vi "Teleop.vi"(10 "Match Info":T1={"Autonomous Elapsed Seconds"=0.0, "TeleOp Elapsed Seconds"=0.0, "Disabled Elapsed Seconds"=0.0, "Visited Autonomous"=FALSE, "Visited TeleOp"=FALSE, "Visited Disabled"=FALSE, "Autonomous Settings"={"Autonomous Style"=enum."Independent", "VI Refnum"=refnum}}, 11 "Call Context":T2) -> ()   [LabVIEW 2014]
doc: "This VI is called for each TeleOp packet received from the DS where the robot is not disabled. It is often used to read from the joysticks and update I/O or to update setpoints for timed control loops. It should complete and return within 20 milliseconds or it may miss DS packets."
uses:
  <vilib>/Rock Robotics/WPI/DriverStation/WPI_DriverStationDerivedRobotMode.ctl
  <vilib>/Rock Robotics/WPI/DriverStation/WPI_DriverStationMatch Info.ctl
  <vilib>/Rock Robotics/WPI/Joystick/WPI_JoystickGetSetRefNum.vi
  Robot Global Data.vi
panel:
  out "Operator Buttons":bool[](array[boolean])
  out "Driver Axis":dbl[](array[numeric])
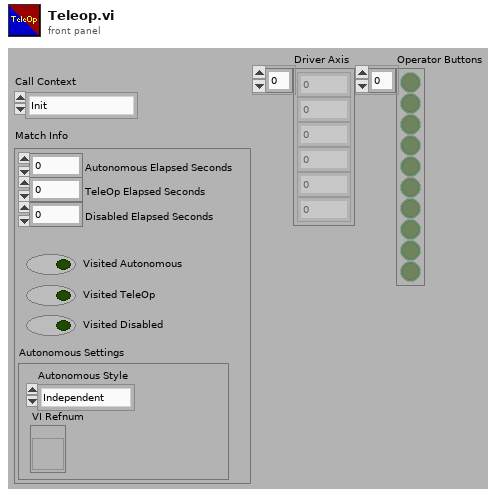
[diagram p1: front panel]
types:
  T1 = typedef "WPI_DriverStationMatch Info.ctl" = cluster{"Autonomous Elapsed Seconds":dbl, "TeleOp Elapsed Seconds":dbl, "Disabled Elapsed Seconds":dbl, "Visited Autonomous":bool, "Visited TeleOp":bool, "Visited Disabled":bool, "Autonomous Settings":cluster{"Autonomous Style":enum16{"Iterative", "Independent"}, "VI Refnum":refnum<vi>}}
  T2 = typedef "WPI_DriverStationDerivedRobotMode.ctl" = enum16{"Init", "Execute", "Stop"}
  T3 = typedef "WPI_JoystickDevRef.ctl" = cluster{"Device":T4}
  T4 = typedef "WPI_JoystickDeviceEnum.ctl" = enum16{"USB 0", "USB 1", "USB 2", "USB 3", "USB 4", "USB 5"}
  T5 = cluster{"String Potentiometer":dbl, "Setpoint":dbl, "Level":sgl}
  T6 = cluster{"Motor Speed":dbl, "Grabber":bool, "Brake":bool, "Trying To Brake":bool}
  T7 = cluster{"Lifter":bool, "Infeeds On":bool, "Descender":bool}
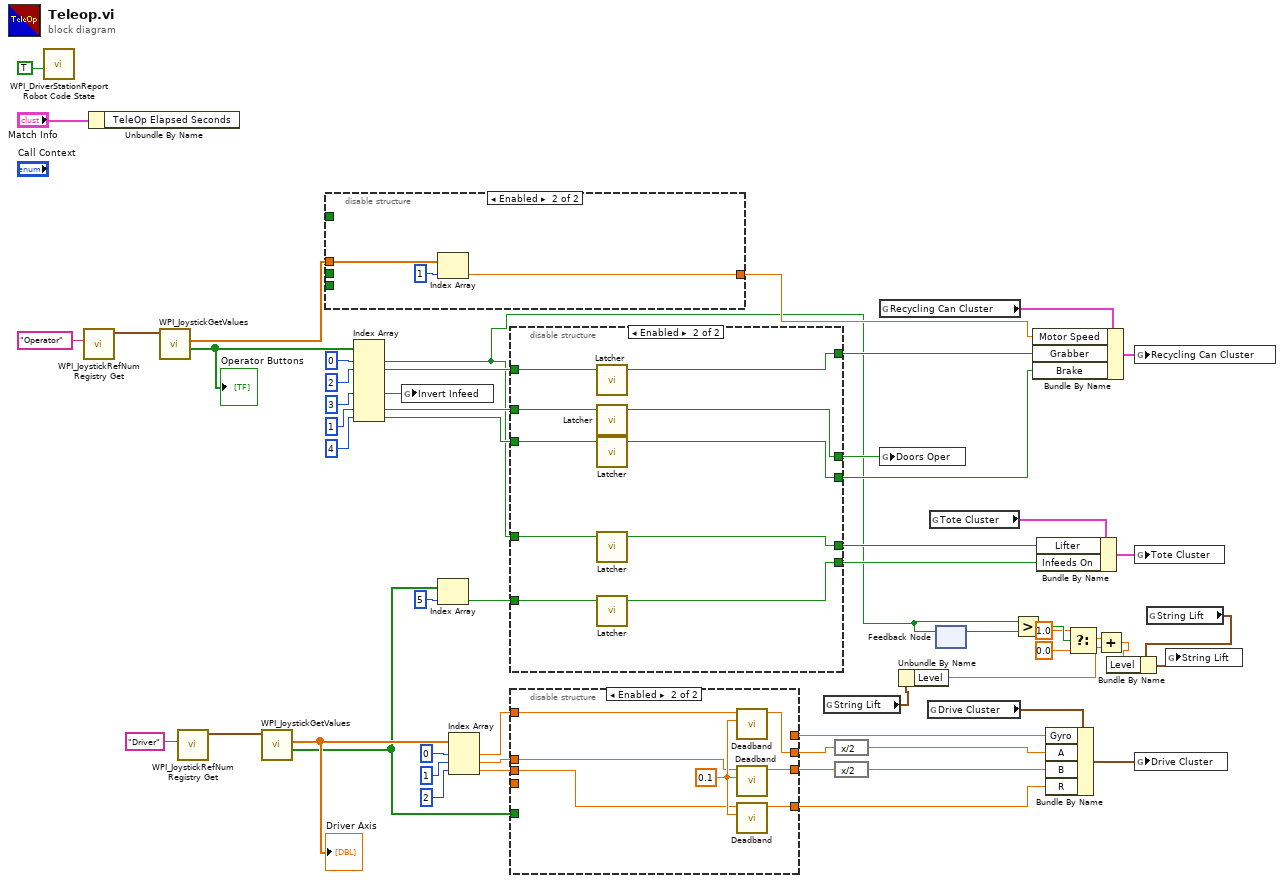
[diagram p0: block diagram]
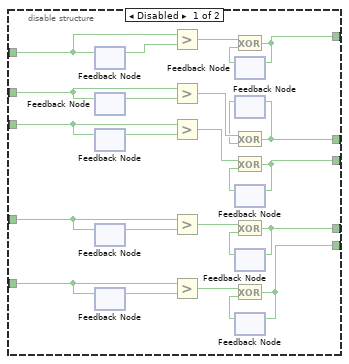
[diagram p2: hidden frame]
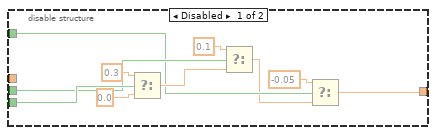
[diagram p3: hidden frame]
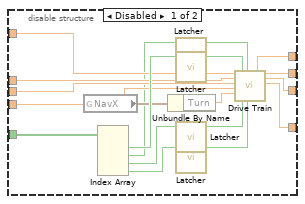
[diagram p4: hidden frame]
diagram:
  n1 = call <vilib>:"WPI_DriverStationReport Robot Code State.vi"("TeleOp"=TRUE ("Autonomous")) -> ()  [unwired: 10 in, 1 out]
  n2 = call <vilib>:"WPI_JoystickRefNum Registry Get.vi"("refnum name"="Operator") -> ("JoystickDevRef"=w42:T3)  [unwired: 9 in, 1 out]
  n3 = Unbundle By Name("Match Info") -> ()  [unwired: 1 out]
  n4 = call <vilib>:"WPI_JoystickGetValues.vi"("JoystickDevRef"=w42) -> ("Buttons"=w39:bool[], "Axes"=w30:dbl[])  [unwired: 6 in, 3 out]
  "Operator Buttons" <- w39
  n5 = call <vilib>:"WPI_JoystickRefNum Registry Get.vi"("refnum name"="Driver") -> ("JoystickDevRef"=w53:T3)  [unwired: 9 in, 1 out]
  n6 = call <vilib>:"WPI_JoystickGetValues.vi"("JoystickDevRef"=w53) -> ("Buttons"=w19:bool[], "Axes"=w21:dbl[])  [unwired: 6 in, 3 out]
  "Driver Axis" <- w21
  n7 = disable-structure shown="Enabled" {
    disable-tunnel: _ -> [w66 _]
    disable-tunnel: _ -> [w61 _]
    disable-tunnel: _ -> [w60 _]
    disable-tunnel: [w58 w67] -> w33
    disable-tunnel: w30 -> [_ w69]
    frame Disabled {
      n8 = Select(t=0.3, s=w66, f=0.0) -> (s? t:f=w63:dbl)
      n9 = Select(t=0.1, s=w61, f=w63) -> (s? t:f=w59:dbl)
      n10 = Select(t=-0.05, s=w60, f=w59) -> (s? t:f=w58:dbl)
    }
    frame Enabled {
      n11 = Index Array(array=w69, index=1) -> (element=w67:dbl)
    }
  }
  n12 = Index Array(array=w39, index #1=0 ("index"), index #2=2 ("index"), index #5=3 ("index"), index #7=1 ("index"), index #8=4 ("index")) -> (element #1=w10:bool, element #2=w17:bool, element #5=w12:bool, element #7=w15:bool, element #8=w16:bool)  [unwired: 3 in, 3 out]
  n13 = global write "Robot Global Data.vi" "Invert Infeed"(w12) -> ()
  n14 = Index Array(array=w19, index=5) -> (element=w18:bool)
  n15 = Index Array(array=w21, index #1=0 ("index"), index #2=1 ("index"), index #3=2 ("index")) -> (element #1=w50:dbl, element #2=w49:dbl, element #3=w48:dbl)
  n16 = disable-structure shown="Enabled" {
    disable-tunnel: [w88 w103] -> w34
    disable-tunnel: [w87 w97] -> w31
    disable-tunnel: [w83 w101] -> w29
    disable-tunnel: [w79 w95] -> w27
    disable-tunnel: w18 -> [w77 w96]
    disable-tunnel: w17 -> [w78 w104]
    disable-tunnel: w16 -> [w76 w102]
    disable-tunnel: w10 -> [w75 w98]
    disable-tunnel: w15 -> [w71 w100]
    disable-tunnel: [w70 w99] -> w14
    frame Disabled {
      n17 = feedback-in #1(w78) -> ()
      n18 = feedback #1() -> (w94:bool)  [unwired: 1 in]
      n19 = feedback #2() -> (w73:bool)  [unwired: 1 in]
      n20 = feedback-in #2(w71) -> ()
      n21 = feedback #3() -> (w86:bool)  [unwired: 1 in]
      n22 = feedback-in #3(w76) -> ()
      n23 = feedback #4() -> (w91:bool)  [unwired: 1 in]
      n24 = feedback-in #4(w75) -> ()
      n25 = feedback #5() -> (w80:bool)  [unwired: 1 in]
      n26 = feedback-in #5(w77) -> ()
      n27 = Greater?(x=w78, y=w94) -> (0:w92:bool)
      n28 = Greater?(x=w71, y=w73) -> (0:w74:bool)
      n29 = Greater?(x=w76, y=w86) -> (0:w84:bool)
      n30 = Greater?(x=w75, y=w91) -> (0:w89:bool)
      n31 = Greater?(x=w77, y=w80) -> (0:w82:bool)
      n32 = feedback #6() -> (w93:bool)  [unwired: 1 in]
      n33 = Exclusive Or(1:w93, 2:w92) -> (0:w88:bool)
      n34 = feedback-in #6(w88) -> ()
      n35 = feedback #7() -> (w72:bool)  [unwired: 1 in]
      n36 = Exclusive Or(1:w72, 2:w74) -> (0:w70:bool)
      n37 = feedback-in #7(w70) -> ()
      n38 = feedback #8() -> (w85:bool)  [unwired: 1 in]
      n39 = Exclusive Or(1:w85, 2:w84) -> (0:w83:bool)
      n40 = feedback-in #8(w83) -> ()
      n41 = feedback #9() -> (w90:bool)  [unwired: 1 in]
      n42 = Exclusive Or(1:w90, 2:w89) -> (0:w87:bool)
      n43 = feedback-in #9(w87) -> ()
      n44 = feedback #10() -> (w81:bool)  [unwired: 1 in]
      n45 = Exclusive Or(1:w81, 2:w82) -> (0:w79:bool)
      n46 = feedback-in #10(w79) -> ()
    }
    frame Enabled {
      n47 = call "Latcher.vi"("Value In"=w104) -> ("Latched"=w103:bool)  [unwired: 4 in]
      n48 = call "Latcher.vi"("Value In"=w100) -> ("Latched"=w99:bool)  [unwired: 4 in]
      n49 = call "Latcher.vi"("Value In"=w102) -> ("Latched"=w101:bool)  [unwired: 4 in]
      n50 = call "Latcher.vi"("Value In"=w98) -> ("Latched"=w97:bool)  [unwired: 4 in]
      n51 = call "Latcher.vi"("Value In"=w96) -> ("Latched"=w95:bool)  [unwired: 4 in]
    }
  }
  n52 = disable-structure shown="Enabled" {
    disable-tunnel: [w123 w130] -> w26
    disable-tunnel: [w122 w128] -> w25
    disable-tunnel: [w121 w127] -> w24
    disable-tunnel: w19 -> [w120 _]
    disable-tunnel: w50 -> [w112 w126]
    disable-tunnel: w49 -> [w111 w125]
    disable-tunnel: w48 -> [w110 w124]
    disable-tunnel: _ -> [w109 _]
    disable-tunnel: [w108 _] -> w47
    frame Disabled {
      n53 = global read "Robot Global Data.vi" "NavX"() -> (w114:cluster{"Update Speed (Hz)":dbl, "Turn":dbl})
      n54 = Index Array(array=w120) -> (element #1=w119:bool, element #2=w106:bool, element #3=w118:bool, element #4=w117:bool)  [unwired: 4 in]
      n55 = Unbundle By Name(w114) -> ("Turn"=w113:dbl)
      n56 = call "Latcher.vi"("Value In"=w106) -> ("Latched"=w105:bool)  [unwired: 4 in]
      n57 = call "Latcher.vi"("Value In"=w119) -> ("Latched"=w107:bool)  [unwired: 4 in]
      n58 = call "Latcher.vi"("Value In"=w118) -> ("Latched"=w115:bool)  [unwired: 4 in]
      n59 = call "Latcher.vi"("Value In"=w117) -> ("Latched"=w116:bool)  [unwired: 4 in]
      n60 = call "Drive Train.vi"("C"=w112, "D"=w111, "X"=w110, "Y"=w109, "gyro"=w113, "Mode Switch"=w107, "Positive 1"=w115, "Turning Switch"=w105, "Negative 1"=w116) -> ("gyro angle"=w108:dbl, "A"=w123:dbl, "B"=w122:dbl, "R"=w121:dbl)  [unwired: 7 in]
    }
    frame Enabled {
      w129 = 0.1 ("y")
      n61 = call "Deadband.vi"("Deadband"=w129, "Motor Speed"=w126) -> ("Power Out"=w130:dbl)  [unwired: 9 in]
      n62 = call "Deadband.vi"("Deadband"=w129, "Motor Speed"=w125) -> ("Power Out"=w128:dbl)  [unwired: 9 in]
      n63 = call "Deadband.vi"("Deadband"=w129, "Motor Speed"=w124) -> ("Power Out"=w127:dbl)  [unwired: 9 in]
    }
  }
  n64 = global read "Robot Global Data.vi" "String Lift"() -> (w6:T5)
  n65 = expression code="x/2"(w26) -> (w22:dbl)
  n66 = expression code="x/2"(w25) -> (w23:dbl)
  n67 = global read "Robot Global Data.vi" "Recycling Can Cluster"() -> (w41:T6)
  n68 = global write "Robot Global Data.vi" "Doors Oper"(w14) -> ()
  n69 = Unbundle By Name(w6) -> ("Level"=w2:sgl)
  n70 = global read "Robot Global Data.vi" "Drive Cluster"() -> (w52:cluster{"A":dbl, "B":dbl, "R":dbl, "Gyro":dbl})
  n71 = global read "Robot Global Data.vi" "Tote Cluster"() -> (w38:T7)
  n72 = feedback #11() -> (w11:bool)  [unwired: 1 in]
  n73 = feedback-in #11(w10) -> ()
  n74 = Greater?(x=w10, y=w11) -> (0:w9:bool)
  n75 = Bundle By Name(cluster=w41, "Motor Speed"=w33, "Grabber"=w34, "Brake"=w29) -> (w40:T6)
  n76 = Bundle By Name(cluster=w38, "Lifter"=w31, "Infeeds On"=w27) -> (w37:T7)
  n77 = Bundle By Name(cluster=w52, "Gyro"=w47, "A"=w22, "B"=w23, "R"=w24) -> (w51:cluster{"A":dbl, "B":dbl, "R":dbl, "Gyro":dbl})
  n78 = Select(t=1.0, s=w9, f=0.0) -> (s? t:f=w3:dbl)
  n79 = Add(x=w3, y=w2) -> (x+y=w1:dbl)
  n80 = global write "Robot Global Data.vi" "Recycling Can Cluster"(w40) -> ()
  n81 = global write "Robot Global Data.vi" "Tote Cluster"(w37) -> ()
  n82 = global write "Robot Global Data.vi" "Drive Cluster"(w51) -> ()
  n83 = global read "Robot Global Data.vi" "String Lift"() -> (w8:T5)
  n84 = Bundle By Name(cluster=w8, "Level"=w1) -> (w7:T5)
  n85 = global write "Robot Global Data.vi" "String Lift"(w7) -> ()
